vi "Process.vi"(8 "error in":errorcluster, 11 "Plugin in":refnum<class "PXIe4113 DUT Power Control Replacement.lvclass">) -> (0 "error out":errorcluster, 3 "Plugin out":refnum<class "PXIe4113 DUT Power Control Replacement.lvclass">)   [LabVIEW 2026, in "PXIe4113 DUT Power Control Replacement.lvlib" / "PXIe4113 DUT Power Control Replacement.lvclass"]
uses:
  PXIe4113 DUT Power Control Replacement.lvclass
  C:/Program Files/National Instruments/LabVIEW 2026/vi.lib/FlexLogger/SDK/PluginSDK.lvlibp/PEFClasses/SDK/Plugin/Plugin.lvclass
  PXIe4113 DUT Power Control Replacement.lvclass/PXIe4113 DUT Power Control Replacement.ctl
  <vilib>/FlexLogger/SDK/PluginSDK.lvlibp/PEFClasses/SDK/Plugin/DataHelpers/Write 1D DBL (NChan 1Sample).vi
  C:/Program Files/National Instruments/LabVIEW 2026/vi.lib/FlexLogger/SDK/PluginSDK.lvlibp/PEFClasses/SDK/Processing Element/Processing Element.lvclass
  C:/Users/localadmin/Documents/LabVIEW Projects/FlexLogger IO Plug-ins/PXIe4113 DUT Power Control Replacement/PXIe4113 DUT Power Control Replacement.lvclass
  <vilib>/FlexLogger/SDK/PluginSDK.lvlibp/PEFClasses/SDK/Plugin/Plugin.lvclass
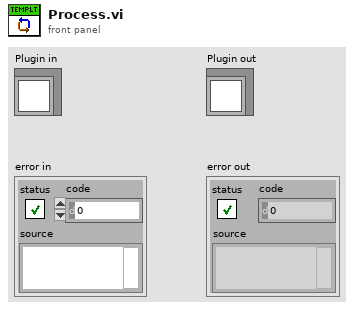
[diagram p1: front panel]
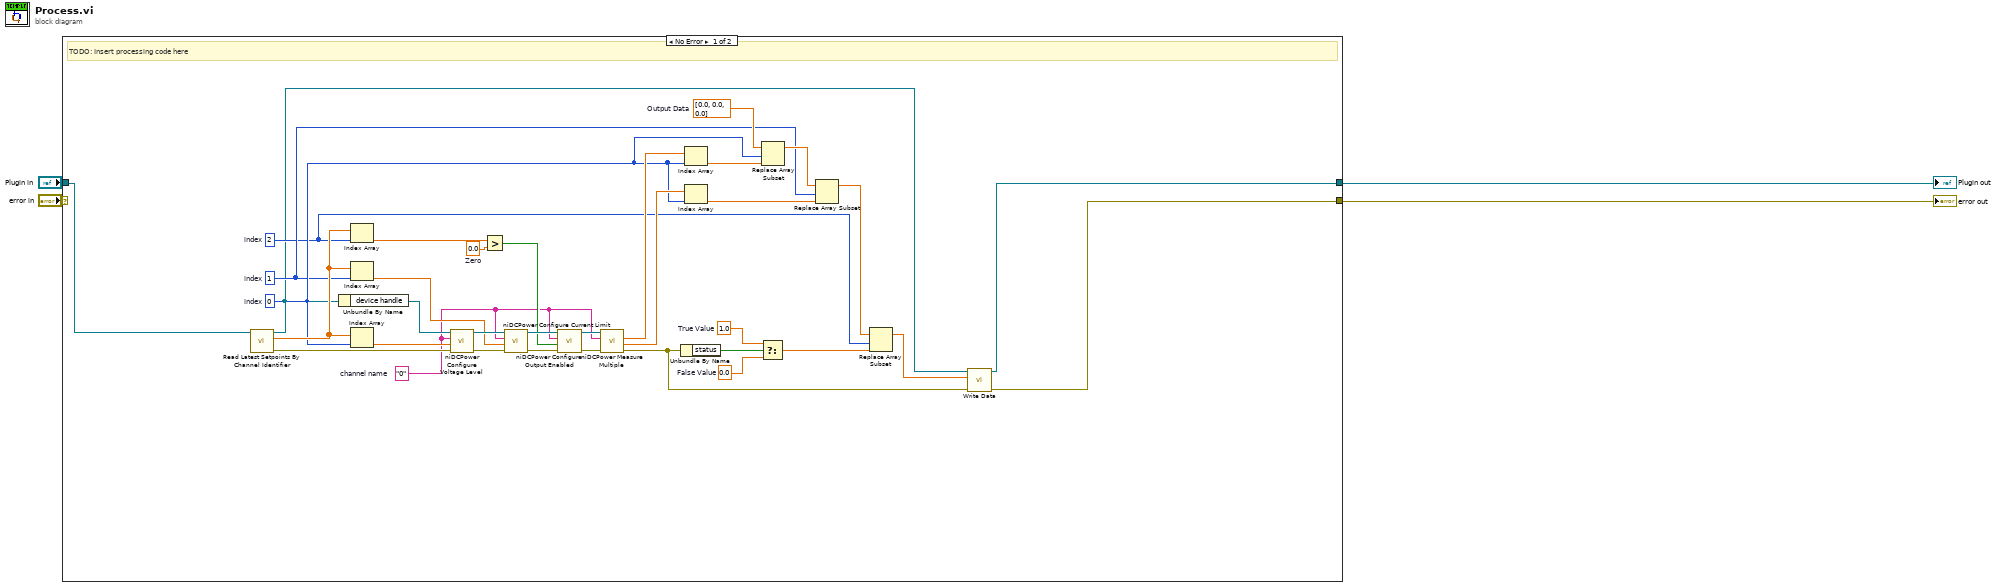
[diagram p0: block diagram]
diagram:
  n1 = case shown="No Error" "error in" {
    selector: "error in" -> [_ w40]
    tunnel: [w6 w41] -> w4
    tunnel: "Plugin in" -> [w39 w41]
    tunnel: [w5 w40] -> w1
    frame No Error {
      w18 = dbl[] [0.0, 0.0, 0.0]  # Output Data
      w19 = 0.0  # False Value
      w21 = 1.0  # True Value
      w30 = 0.0  # Zero
      w11 = 2  # index
      w14 = 1  # index
      w17 = 0  # index
      w25 = "0"  # channel name
      # "TODO: Insert processing code here"
      n2 = call <vilib>:"Read Latest Setpoints By Channel Identifier.vi"("Plugin in"=w39) -> ("error out"=w35:errorcluster, "Channel Setpoints"=w38:dbl[], "Plugin out"=w9:refnum<class "PXIe4113 DUT Power Control Replacement.lvclass">)  [unwired: 7 in, 1 out]
      n3 = Unbundle By Name(w9) -> ("device handle"=w37:refnum<k15>)
      n4 = Index Array(array=w38, index=w11) -> (element=w31:dbl)
      n5 = Index Array(array=w38, index=w14) -> (element=w33:dbl)
      n6 = Index Array(array=w38, index=w17) -> (element=w36:dbl)
      n7 = call <instrlib>:"niDCPower Configure Voltage Level.vi"("error in (no error)"=w35, "voltage level"=w36, "channel name"=w25, "instrument handle"=w37) -> ("error out"=w32:errorcluster, "instrument handle out"=w34:refnum<k15>)  [unwired: 6 in]
      n8 = Greater?(x=w31, y=w30) -> (0:w28:bool)
      n9 = call <instrlib>:"niDCPower Configure Current Limit.vi"("error in (no error)"=w32, "current limit"=w33, "channel name"=w25, "instrument handle"=w34) -> ("error out"=w27:errorcluster, "instrument handle out"=w29:refnum<k15>)  [unwired: 6 in]
      n10 = call <instrlib>:"niDCPower Configure Output Enabled.vi"("error in (no error)"=w27, "output enabled"=w28, "channel name"=w25, "instrument handle"=w29) -> ("error out"=w24:errorcluster, "instrument handle out"=w26:refnum<k15>)  [unwired: 6 in]
      n11 = call <instrlib>:"niDCPower Measure Multiple.vi"("error in (no error)"=w24, "channel name"=w25, "instrument handle"=w26) -> ("error out"=w7:errorcluster, "current measurements"=w22:dbl[], "voltage measurements"=w23:dbl[])  [unwired: 5 in, 1 out]
      n12 = Unbundle By Name(w7) -> ("status"=w20:bool)
      n13 = Index Array(array=w23, index=w17) -> (element=w16:dbl)
      n14 = Index Array(array=w22, index=w17) -> (element=w13:dbl)
      n15 = Select(t=w21, s=w20, f=w19) -> (s? t:f=w10:dbl)
      n16 = Replace Array Subset(array=w18, new element=w16, index=w17) -> (w15:dbl[])
      n17 = Replace Array Subset(array=w15, new element=w13, index=w14) -> (w12:dbl[])
      n18 = Replace Array Subset(array=w12, new element=w10, index=w11) -> (w8:dbl[])
      n19 = call-poly <vilib>:"Write Data.vi"("error in (no error)"=w7, "Data"=w8, "Plugin in"=w9) -> ("error out"=w5:errorcluster, "Plugin out"=w6:refnum<class "PXIe4113 DUT Power Control Replacement.lvclass">)  [unwired: 7 in]
    }
    frame Error {
    }
  }
  "error out" <- w1
  "Plugin out" <- w4
